vi "Vettori lezione.vi"() -> ()   [LabVIEW 2012]
doc: "M. Ferrari - M. Corti"
panel:
  in  "N° comp.":i32=4
  in  "Init value":sgl=2.0 format="%.2f"
  out "array2":sgl[](array[numeric]) format="%.2f"
  out "array1":sgl[](array[numeric]) format="%.2f"
  out "Vet som":i32[](array[numeric])
  in  "vet b":i32[](array[numeric])=[0, 0, 4, 4, 2]
  in  "vet a":i32[](array[numeric])=[0, 2, -2, 4, -5]
  in  "select":u16(ring) items=["Ciclo WHILE", "Ciclo FOR"]
  in  "n° comp. 1":i32=2
  out "vet 1":dbl[](array[numeric]) format="%.2f"
  # "CREAZIONE AUTOMATICA di un VETTORE"
  # "Inizializzazione degli array"
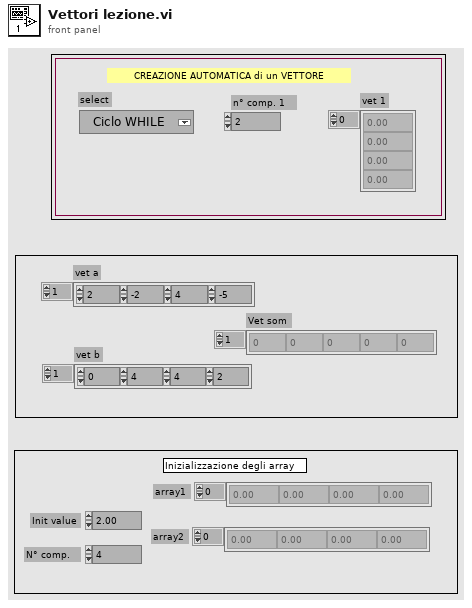
[diagram p1: front panel]
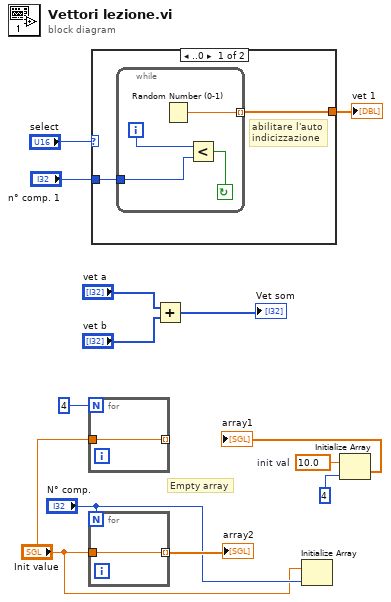
[diagram p0: block diagram]
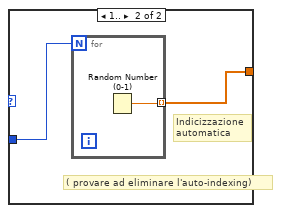
[diagram p2: hidden frame]
diagram:
  w6 = sgl 10.0  # init val
  # "Empty array"
  n1 = for {
    N: 4 -> [_]
    tunnel: "Init value" -> [w14]
    tunnel: [w14] -> _ mode=indexing
  }
  n2 = for {
    N: "N° comp." -> [_]
    tunnel: "Init value" -> [w15]
    tunnel: [w15] -> w4 mode=indexing
  }
  "array2" <- w4
  n3 = case shown="..0" "select" {
    tunnel: [w17 w22] -> w12
    tunnel: "n° comp. 1" -> [w16 w23]
    frame ..0 {
      # "abilitare l'auto\nindicizzazione"
      n4 = while {
        tunnel: [w21] -> w17 mode=indexing
        tunnel: w16 -> [w20]
        i -> [w19]
        stop <- w18 continue-if-true
        n5 = Random Number (0-1)() -> (number: 0 to 1=w21:dbl)
        n6 = Less?(x=w19, y=w20) -> (x < y?=w18:bool)
      }
    }
    frame 1.. {
      # "( provare ad eliminare l'auto-indexing)"
      # "Indicizzazione\nautomatica"
      n7 = for {
        N: w23 -> [_]
        tunnel: [w24] -> w22 mode=indexing
        n8 = Random Number (0-1)() -> (number: 0 to 1=w24:dbl)
      }
    }
  }
  "vet 1" <- w12
  n9 = Add(x="vet a", y="vet b") -> (x+y=→"Vet som":i32[])
  n10 = Initialize Array("Init value", "N° comp.") -> ()  [unwired: 1 out]
  n11 = Initialize Array(w6, 4) -> (→"array1":sgl[])
